vi "Read Packet.vi"(11 "Packet Msg in":refnum<class "Packet Msg.lvclass">) -> (2 "Packet":string, 3 "Packet Msg out":refnum<class "Packet Msg.lvclass">)   [LabVIEW 2015, in "TCPIP Communications Framework.lvlib" / "Packet Msg.lvclass"]
uses:
  Packet Msg.lvclass
  Packet Msg.lvclass/Packet Msg.ctl
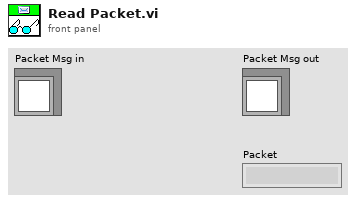
[diagram p1: front panel]
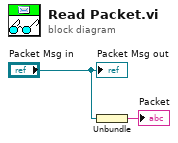
[diagram p0: block diagram]
diagram:
  n1 = Unbundle("Packet Msg in") -> (→"Packet":string)
  "Packet Msg out" <- "Packet Msg in"
